vi "ConfigFEQ - 複製.vi"(8 "error in (no error)":errorcluster, 10 "Frequency (1:1kHz)":u16(ring)=1 items=["120 Hz Frequency", "1 kHz Frequency", "1 MHz Frequency"], 11 "VISA resource name":refnum<visa-resource-name>) -> (0 "error out":errorcluster, 3 "VISA resource name out":refnum<visa-resource-name>)   [LabVIEW 2012]
panel:
  in  "Frequency Shift (2: 0%)":u16(ring)=2 items=["-2%", "-1%", "0%", "1%", "2%"]
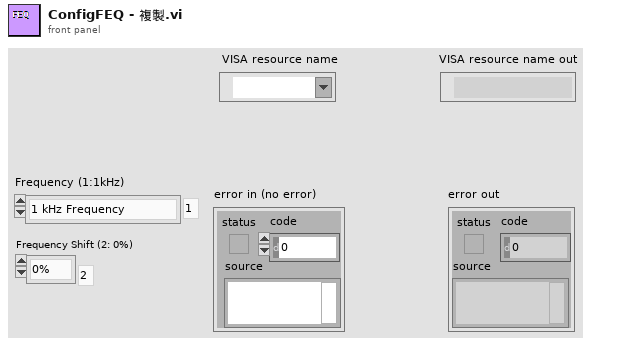
[diagram p1: front panel]
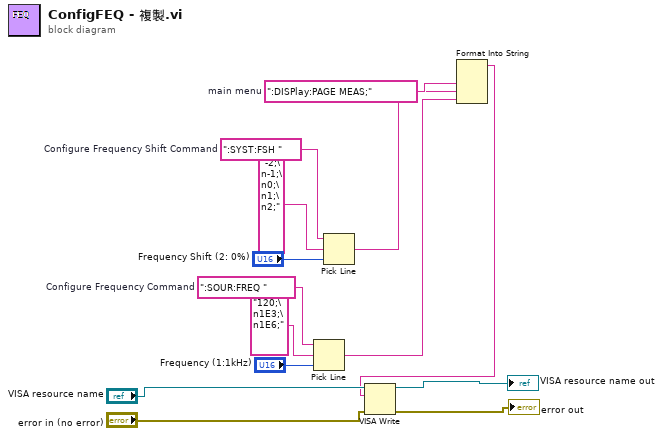
[diagram p0: block diagram]
diagram:
  w6 = ":DISPlay:PAGE MEAS;"  # main menu
  w10 = ":SYST:FSH "  # Configure Frequency Shift Command
  w11 = ":SOUR:FREQ "  # Configure Frequency Command
  n1 = Pick Line(string ("")=w11, multi-line string="120;\n1E3;\n1E6;", line index="Frequency (1:1kHz)") -> (output string=w4:string)
  n2 = Pick Line(string ("")=w10, multi-line string="-2;\n-1;\n0;\n1;\n2;", line index="Frequency Shift (2: 0%)") -> (output string=w5:string)
  n3 = Format Into String(w6, w5, w4) -> (resulting string=w1:string)  [unwired: 3 in, 1 out]
  n4 = VISA Write(VISA resource name="VISA resource name", write buffer=w1, error in (no error)="error in (no error)") -> (VISA resource name out=→"VISA resource name out":refnum<visa-resource-name>, error out=→"error out":errorcluster)  [unwired: 1 out]
